vi "Close.vi"(8 "Error In":errorcluster, 11 "SDO Manager":refnum<class "SDO Manager.lvclass">) -> (0 "Error Out":errorcluster, 3 "SDO Manager":refnum<class "SDO Manager.lvclass">)   [LabVIEW 2020, in "SDO Manager.lvlib" / "SDO Manager.lvclass"]
uses:
  SDO Manager.lvclass/SDO Manager.ctl
  SDO Manager.lvclass
  <vilib>/ActorFramework/Stop Msg/Stop Msg.lvclass
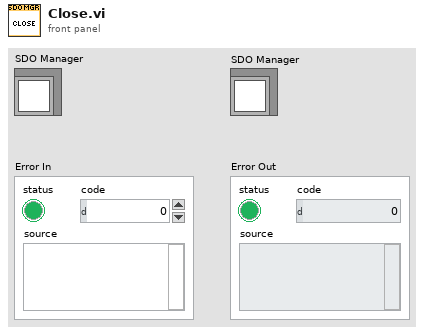
[diagram p1: front panel]
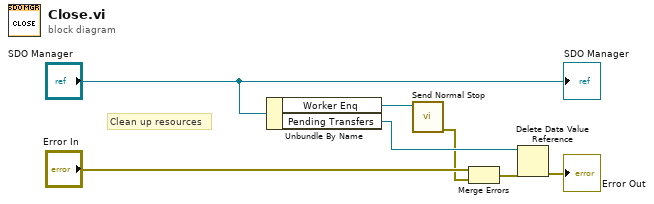
[diagram p0: block diagram]
diagram:
  # "Clean up resources"
  n1 = Unbundle By Name("SDO Manager") -> ("Worker Enq"=w5:refnum<class "Message Enqueuer.lvclass">, "Pending Transfers"=w7:refnum<data-value>)
  n2 = call <vilib>:"Send Normal Stop.vi"("Message Enqueuer"=w5) -> ("error out"=w1:errorcluster)  [unwired: 10 in]
  n3 = Merge Errors("Error In", w1) -> (w3:errorcluster)
  n4 = Delete Data Value Reference(data value reference=w7, error in=w3) -> (error out=→"Error Out":errorcluster)  [unwired: 1 out]
  "SDO Manager" <- "SDO Manager"
